vi "SetState.vi"(8 "Error In":errorcluster, 10 "State":bool, 11 "reference in":refnum<class "VdDigitalControl_Simulated.lvclass">) -> (0 "Error Out":errorcluster, 3 "reference out":refnum<class "VdDigitalControl_Simulated.lvclass">)   [LabVIEW 2020, in "VdDigitalControl_Simulated.lvclass"]
uses:
  VdDigitalControl_Simulated.lvclass
  VdDigitalControl_class/VdDigitalControl.lvclass
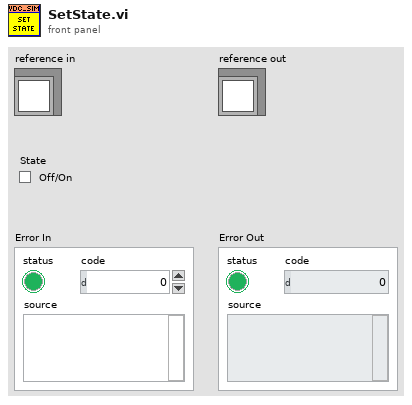
[diagram p1: front panel]
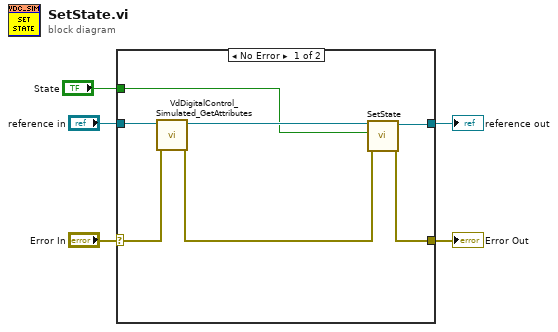
[diagram p0: block diagram]
diagram:
  n1 = case shown="No Error" "Error In" {
    selector: "Error In" -> [w7 w14]
    tunnel: [w9 w14] -> w4
    tunnel: [w10 w13] -> w2
    tunnel: "reference in" -> [w12 w13]
    tunnel: "State" -> [w8 _]
    frame No Error {
      n2 = call "VdDigitalControl_Simulated_GetAttributes.vi"("error in (no error)"=w7, "reference in"=w12) -> ("error out"=w6:errorcluster, "reference out"=w11:refnum<class "VdDigitalControl_Simulated.lvclass">)  [unwired: 6 in, 2 out]
      n3 = call-parent "SetState.vi"("Error In"=w6, "State"=w8, "reference in"=w11) -> ("Error Out"=w9:errorcluster, "reference in"=w10:refnum<class "VdDigitalControl_Simulated.lvclass">)  [unwired: 7 in]
    }
    frame Error {
    }
  }
  "Error Out" <- w4
  "reference out" <- w2
